vi "4461 - AI AND AI - Read AND Write Uneven.vi"(4 "Reset":bool, 6 "AO Array":waveform(dbl)[](array[waveform]), 8 "error in (no error)":errorcluster, 9 "sampling info":cluster{"Fs":dbl, "#s":dbl}={"Fs"=1000.0, "#s"=1000.0} {"Fs" format="%.2p"}, 10 "AO Task":refnum<k21>[](array[refnum]), 11 "AI task":refnum<k21>[](array[refnum])=["", ""]) -> (0 "error out":errorcluster, 3 "Input Signals":waveform(dbl)[](array[waveform]))   [LabVIEW 2013]
uses:
  <vilib>/DAQmx/write.llb/DAQmx Write (Analog 1D Wfm NChan NSamp).vi
  <vilib>/DAQmx/read.llb/DAQmx Read (Analog 1D Wfm NChan NSamp).vi
  <vilib>/DAQmx/miscellaneous.llb/DAQmx Fill In Error Info.vi
  <resource>/objmgr/daqmx.rc
panel:
  out "Numeric":i32
  out "AvailSampPerChan 4":u32
  out "AvailSampPerChan 3":u32
  out "AvailSampPerChan 2":u32
  out "AvailSampPerChan 1":u32
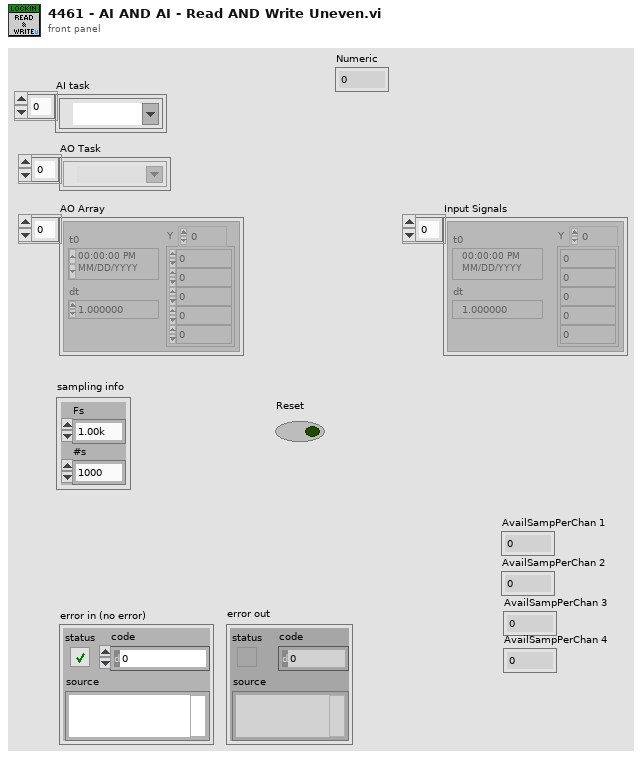
[diagram p1: front panel]
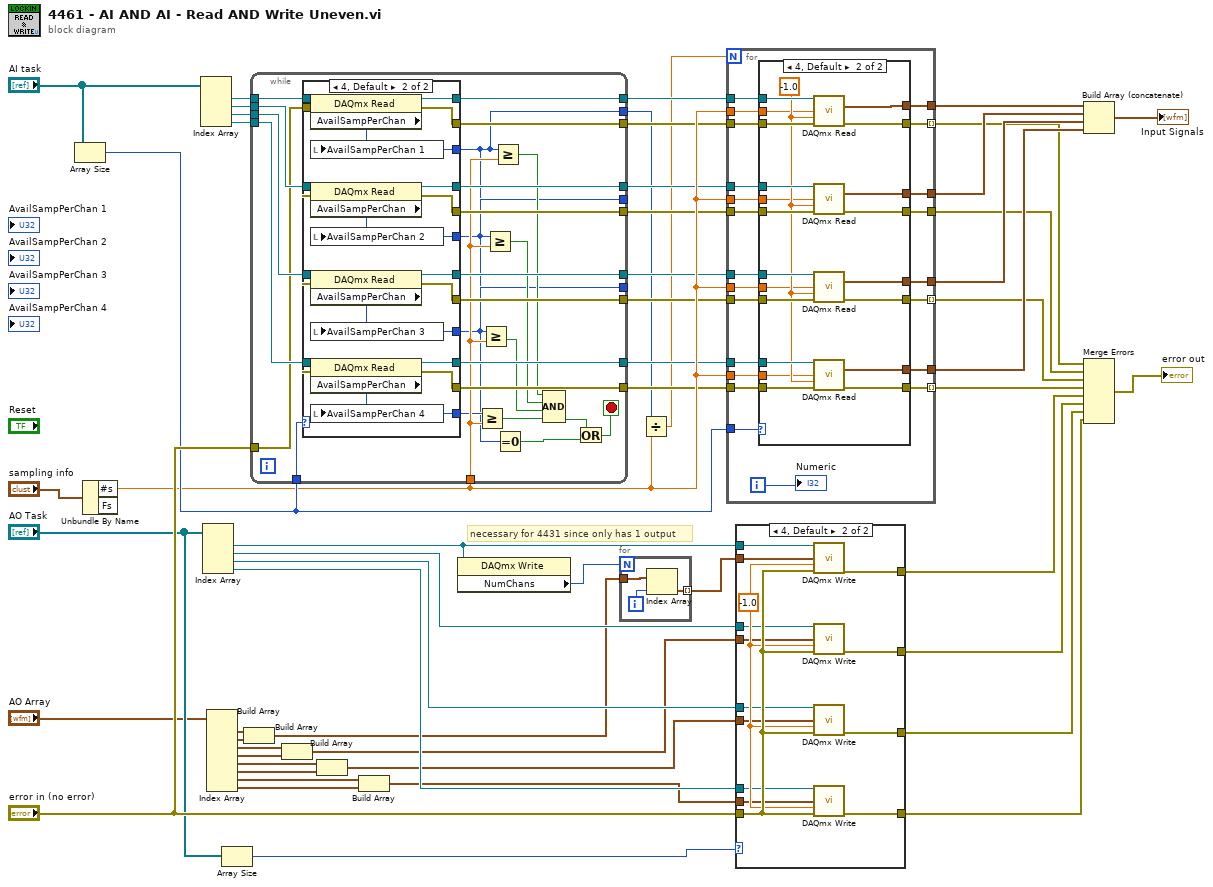
[diagram p0: block diagram]
diagram:
  # "necessary for 4431 since only has 1 output"
  n1 = Array Size(array="AI task") -> (size(s)=w51:i32)
  n2 = Unbundle By Name("sampling info") -> ("#s"=w50:dbl)  [unwired: 1 out]
  n3 = Index Array(array="AI task") -> (element #1=w42:refnum<k21>, element #2=w43:refnum<k21>, element #3=w44:refnum<k21>, element #4=w45:refnum<k21>)  [unwired: 4 in]
  n4 = Index Array(array="AO Task") -> (element #1=w5:refnum<k21>, element #2=w25:refnum<k21>, element #3=w24:refnum<k21>, element #4=w23:refnum<k21>)  [unwired: 4 in]
  n5 = Index Array(array="AO Array") -> (element #1=w26:waveform(dbl), element #2=w27:waveform(dbl), element #3=w28:waveform(dbl), element #4=w29:waveform(dbl), element #5=w30:waveform(dbl), element #6=w31:waveform(dbl), element #7=w32:waveform(dbl), element #8=w33:waveform(dbl))  [unwired: 8 in]
  n6 = Array Size(array="AO Task") -> (size(s)=w1:i32)
  n7 = Build Array(w26, w27) -> (w2:waveform(dbl)[])
  n8 = while {
    tunnel: w45 -> [w80]
    tunnel: w44 -> [w79]
    tunnel: w43 -> [w78]
    tunnel: w42 -> [w77]
    tunnel: [w76] -> w41
    tunnel: [w75] -> w40
    tunnel: [w74] -> w39
    tunnel: [w73] -> w38
    tunnel: "error in (no error)" -> [w68]
    tunnel: [w72] -> w37
    tunnel: [w71] -> w36
    tunnel: [w70] -> w35
    tunnel: [w69] -> w34
    tunnel: w50 -> [w62]
    tunnel: [w57] -> w6
    tunnel: [w59] -> _
    tunnel: [w58] -> _
    tunnel: w51 -> [w56]
    stop <- w61 stop-if-true
    n9 = case shown="4, Default" w56 {
      tunnel: w80 -> [_ w97]
      tunnel: w79 -> [_ w96]
      tunnel: w78 -> [_ w95]
      tunnel: w77 -> [_ w94]
      tunnel: [_ w93] -> w76
      tunnel: [_ w92] -> w75
      tunnel: [_ w91] -> w74
      tunnel: [_ w90] -> w73
      tunnel: [_ w89] -> w72
      tunnel: [_ w88] -> w71
      tunnel: [_ w87] -> w70
      tunnel: [_ w86] -> w69
      tunnel: w68 -> [_ w85]
      tunnel: [_ w84] -> w60
      tunnel: [_ w83] -> w59
      tunnel: [_ w82] -> w58
      tunnel: [_ w81] -> w57
      frame 0 {
      }
      frame 4, Default {
        n10 = property class="DAQmx Read"(reference=w94, error in=w85) -> (reference out=w93:refnum<k21>, error out=w89:errorcluster, "AvailSampPerChan"=w81:u32)
        n11 = local write "AvailSampPerChan 1"(w81) -> ()
        n12 = property class="DAQmx Read"(reference=w95, error in=w85) -> (reference out=w92:refnum<k21>, error out=w88:errorcluster, "AvailSampPerChan"=w82:u32)
        n13 = local write "AvailSampPerChan 2"(w82) -> ()
        n14 = property class="DAQmx Read"(reference=w96, error in=w85) -> (reference out=w91:refnum<k21>, error out=w87:errorcluster, "AvailSampPerChan"=w83:u32)
        n15 = local write "AvailSampPerChan 3"(w83) -> ()
        n16 = property class="DAQmx Read"(reference=w97, error in=w85) -> (reference out=w90:refnum<k21>, error out=w86:errorcluster, "AvailSampPerChan"=w84:u32)
        n17 = local write "AvailSampPerChan 4"(w84) -> ()
      }
    }
    n18 = Greater Or Equal?(x=w60, y=w62) -> (x >= y?=w67:bool)
    n19 = Greater Or Equal?(x=w59, y=w62) -> (x >= y?=w66:bool)
    n20 = Greater Or Equal?(x=w58, y=w62) -> (x >= y?=w65:bool)
    n21 = Greater Or Equal?(x=w57, y=w62) -> (x >= y?=w64:bool)
    n22 = Equal To 0?(x=w57) -> (x = 0?=w55:bool)
    n23 = Compound Arithmetic op=AND(w64, w65, w66, w67) -> (w63:bool)
    n24 = Or(x=w63, y=w55) -> (x .or. y?=w61:bool)
  }
  n25 = Build Array(w28, w29) -> (w22:waveform(dbl)[])
  n26 = Build Array(w30, w31) -> (w21:waveform(dbl)[])
  n27 = Build Array(w32, w33) -> (w20:waveform(dbl)[])
  n28 = property class="DAQmx Write"(reference=w5) -> ("NumChans"=w4:u32)  [unwired: 1 in, 2 out]
  n29 = for {
    N: w4 -> [_]
    tunnel: w2 -> [w100]
    tunnel: [w99] -> w3 mode=indexing
    i -> [w98]
    n30 = Index Array(array=w100, index=w98) -> (element=w99:waveform(dbl))
  }
  n31 = Divide(x=w6, y=w50) -> (x/y=w7:dbl)
  n32 = for {
    N: w7 -> [_]
    tunnel: w41 -> [w122]
    tunnel: w40 -> [w121]
    tunnel: w39 -> [w120]
    tunnel: w38 -> [w119]
    tunnel: w37 -> [w118]
    tunnel: w36 -> [w117]
    tunnel: w35 -> [w116]
    tunnel: w34 -> [w115]
    tunnel: [w114] -> w15
    tunnel: [w113] -> w14
    tunnel: [w112] -> w13
    tunnel: [w111] -> w12
    tunnel: w50 -> [w110]
    tunnel: w50 -> [w109]
    tunnel: w50 -> [w108]
    tunnel: w50 -> [w107]
    tunnel: [w106] -> w11 mode=indexing
    tunnel: [w105] -> w10
    tunnel: [w104] -> w9 mode=indexing
    tunnel: [w103] -> w8 mode=indexing
    tunnel: w51 -> [w101]
    i -> [w102]
    n33 = case shown="4, Default" w101 {
      tunnel: w122 -> [_ w143]
      tunnel: w121 -> [_ w142]
      tunnel: w120 -> [_ w141]
      tunnel: w119 -> [_ w140]
      tunnel: w118 -> [_ w139]
      tunnel: w117 -> [_ w138]
      tunnel: w116 -> [_ w137]
      tunnel: w115 -> [_ w136]
      tunnel: [_ w134] -> w114
      tunnel: [_ w133] -> w113
      tunnel: [_ w132] -> w112
      tunnel: [_ w131] -> w111
      tunnel: w110 -> [_ w130]
      tunnel: w109 -> [_ w129]
      tunnel: w108 -> [_ w128]
      tunnel: w107 -> [_ w127]
      tunnel: [_ w126] -> w106
      tunnel: [_ w125] -> w105
      tunnel: [_ w124] -> w104
      tunnel: [_ w123] -> w103
      frame 0 {
      }
      frame 4, Default {
        w135 = -1.0 ("timeout")
        n34 = call-poly <vilib>:"DAQmx Read.vi"("task/channels in"=w143, "number of samples per channel"=w129, "timeout"=w135, "error in"=w139) -> ("data"=w133:waveform(dbl)[], "error out"=w126:errorcluster)  [unwired: 9 in, 1 out]
        n35 = call-poly <vilib>:"DAQmx Read.vi"("task/channels in"=w142, "number of samples per channel"=w127, "timeout"=w135, "error in"=w138) -> ("data"=w134:waveform(dbl)[], "error out"=w125:errorcluster)  [unwired: 9 in, 1 out]
        n36 = call-poly <vilib>:"DAQmx Read.vi"("task/channels in"=w141, "number of samples per channel"=w128, "timeout"=w135, "error in"=w137) -> ("data"=w132:waveform(dbl)[], "error out"=w124:errorcluster)  [unwired: 9 in, 1 out]
        n37 = call-poly <vilib>:"DAQmx Read.vi"("task/channels in"=w140, "number of samples per channel"=w130, "timeout"=w135, "error in"=w136) -> ("data"=w131:waveform(dbl)[], "error out"=w123:errorcluster)  [unwired: 9 in, 1 out]
      }
    }
    "Numeric" <- w102
  }
  n38 = case shown="4, Default" w1 {
    tunnel: "error in (no error)" -> [_ w157]
    tunnel: w25 -> [_ w155]
    tunnel: w24 -> [_ w154]
    tunnel: w23 -> [_ w153]
    tunnel: w22 -> [_ w152]
    tunnel: w21 -> [_ w151]
    tunnel: w20 -> [_ w150]
    tunnel: [_ w149] -> w19
    tunnel: [_ w148] -> w18
    tunnel: [_ w147] -> w17
    tunnel: [_ w146] -> w16
    tunnel: w5 -> [_ w145]
    tunnel: w3 -> [_ w144]
    frame 0 {
    }
    frame 4, Default {
      w156 = -1.0 ("timeout")
      n39 = call-poly <vilib>:"DAQmx Write.vi"("task/channels in"=w145, "data"=w144, "timeout"=w156, "error in"=w157) -> ("error out"=w149:errorcluster)  [unwired: 9 in, 2 out]
      n40 = call-poly <vilib>:"DAQmx Write.vi"("task/channels in"=w155, "data"=w152, "timeout"=w156, "error in"=w157) -> ("error out"=w148:errorcluster)  [unwired: 9 in, 2 out]
      n41 = call-poly <vilib>:"DAQmx Write.vi"("task/channels in"=w154, "data"=w151, "timeout"=w156, "error in"=w157) -> ("error out"=w147:errorcluster)  [unwired: 9 in, 2 out]
      n42 = call-poly <vilib>:"DAQmx Write.vi"("task/channels in"=w153, "data"=w150, "timeout"=w156, "error in"=w157) -> ("error out"=w146:errorcluster)  [unwired: 9 in, 2 out]
    }
  }
  n43 = Build Array (concatenate)(w14, w15, w13, w12) -> (→"Input Signals":waveform(dbl)[])
  n44 = Merge Errors(w11, w10, w9, w8, w19, w18, w17, w16) -> (→"error out":errorcluster)
